vi "dfd_X Equal Y.vi"   [LabVIEW 2017, in "NI_DigFilterLicensed.lvlib"]
uses:
  <vilib>/addons/Digital Filter Design/NI_DigFilterLicensed.lvlib
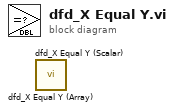
[diagram p0: block diagram]
diagram:
  n1 = call <vilib>:"dfd_X Equal Y (Array).vi"() -> ()  [unwired: 7 in, 1 out]
  n2 = call <vilib>:"dfd_X Equal Y (Scalar).vi"() -> ()  [unwired: 7 in, 1 out]
